vi "wait for fp element value stable.vi"(8 "error in":errorcluster, 11 "CtlRef":refnum<vi>) -> (0 "error out":errorcluster, 3 "Value":variant)   [LabVIEW 2017]
doc: "SciScan 1.2 160622"
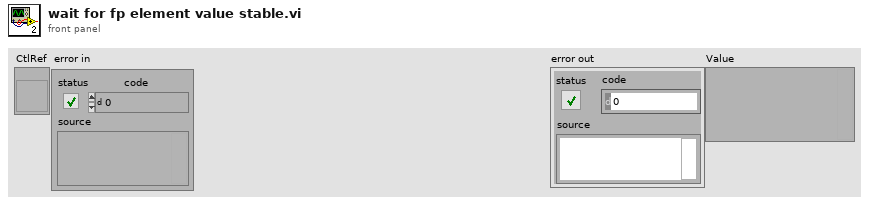
[diagram p1: front panel]
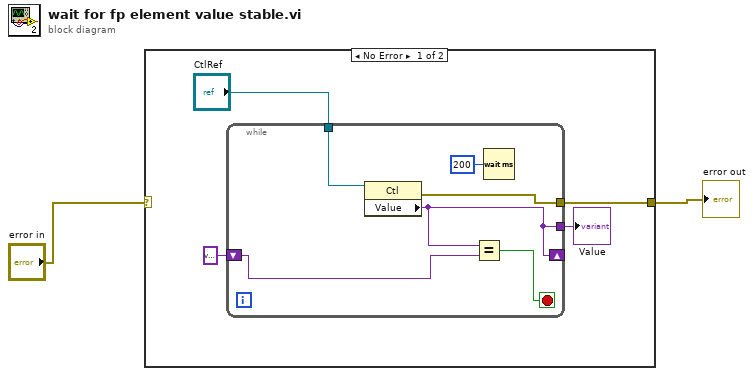
[diagram p0: block diagram]
diagram:
  n1 = case shown="No Error" "error in" {
    selector: "error in" -> [_ w13]
    tunnel: [w5 w13] -> w1
    frame No Error {
      n2 = while {
        tunnel: "CtlRef" -> [w12]
        tunnel: [w9] -> w5
        tunnel: [w7] -> w4
        shift-right: [w7] -> _
        shift-left: variant ("Value") -> [w8]
        stop <- w11 stop-if-true
        n3 = property class="Ctl"(reference=w12) -> (error out=w9:errorcluster, "Value"=w7:variant)  [unwired: 1 in, 1 out]
        n4 = Equal?(x=w7, y=w8) -> (x = y?=w11:bool)
        n5 = Wait (ms)(milliseconds to wait=u32 200) -> ()  [unwired: 1 out]
      }
      "Value" <- w4
    }
    frame Error {
    }
  }
  "error out" <- w1
